vi "DllCall.vi"() -> ()   [LabVIEW 2022 SP3]
uses:
  build/libopendaq-bridge.so
panel:
  out "return type 2":u64
  out "error out":errorcluster
  in  "return type":u64
  in  "error in (no error)":errorcluster
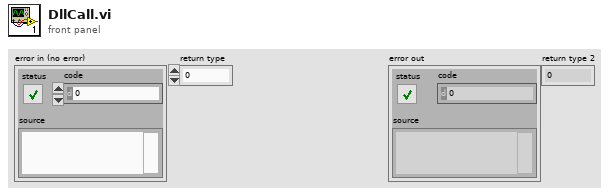
[diagram p1: front panel]
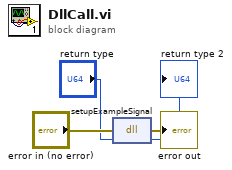
[diagram p0: block diagram]
diagram:
  n1 = dll-call lib="home/vlad/Desktop/opendaq/opendaq-3.0.0-examples/cpp/OpenDAQ-Glue/build/libopendaq-bridge.so" fn="setupExampleSignal"(error in="error in (no error)", "return type"="return type") -> (error out=→"error out":errorcluster, "return type"=→"return type 2":u64)  [unwired: 1 in, 1 out]
